vi "Rework补充.vi"() -> ()   [LabVIEW 2014]
uses:
  <vilib>/addons/database/NI_Database_API.lvlib
  <vilib>/addons/database/Connection.llb/DB Tools Open Connec (String).vi
panel:
  in  "选项卡控件":enum32{"主界面", "监控界面"}(tab)
  in  "退出":bool
  in  "RFID值":string
  in  "确定按钮":bool
  out "修改状态":string
  out "error out":errorcluster
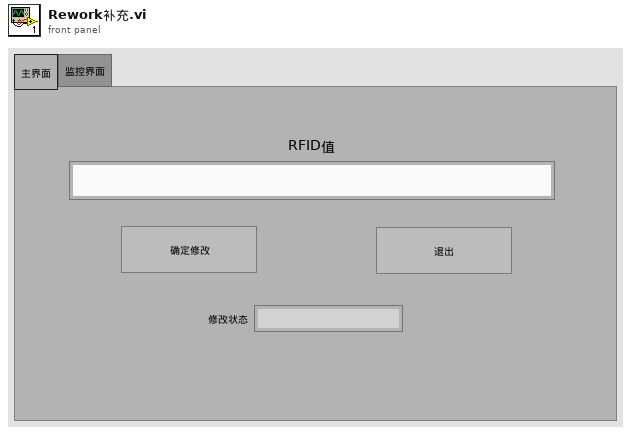
[diagram p1: front panel]
types:
  T1 = typedef "NI_Database_API.lvlib/Conn ObjectReference.ctl" = refnum<k1>
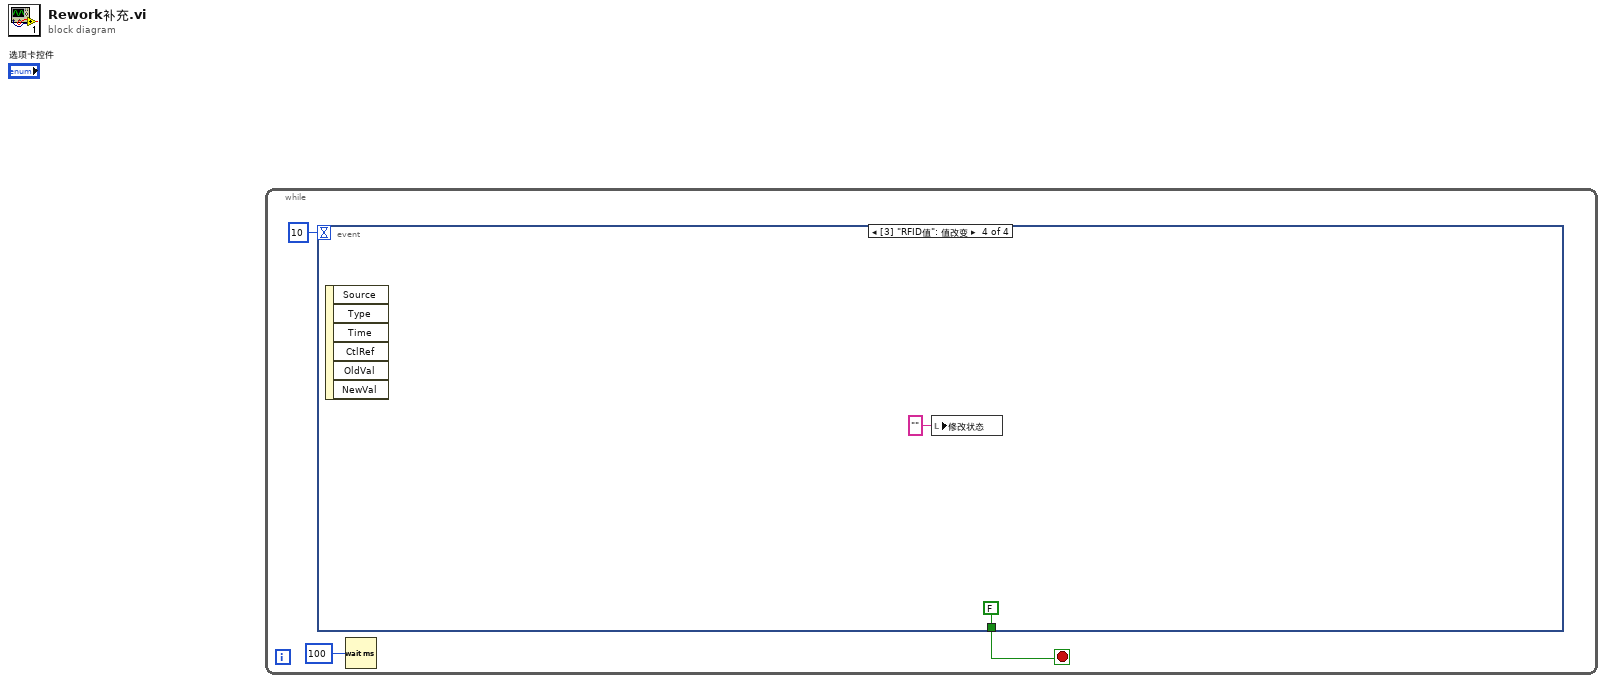
[diagram p0: block diagram]
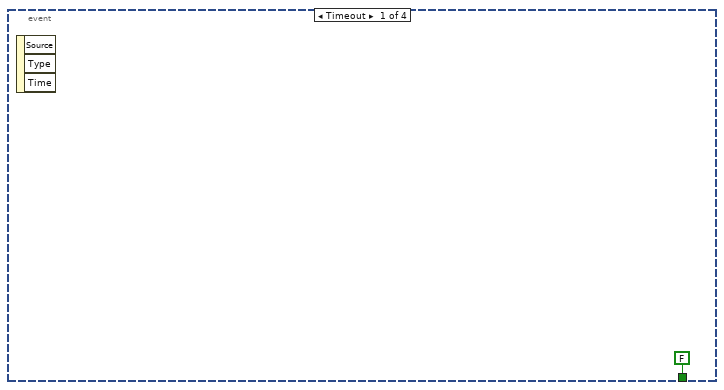
[diagram p2: hidden frame]
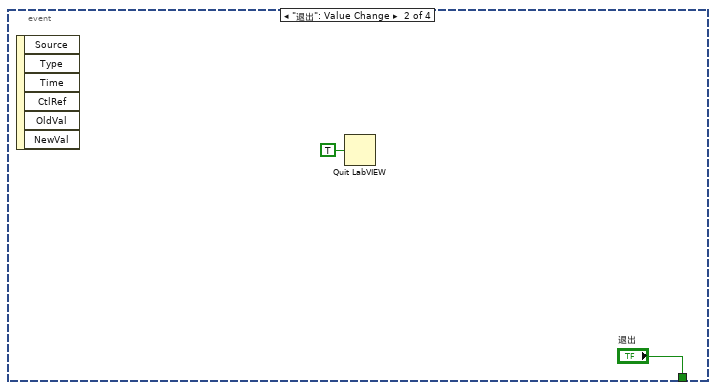
[diagram p3: hidden frame]
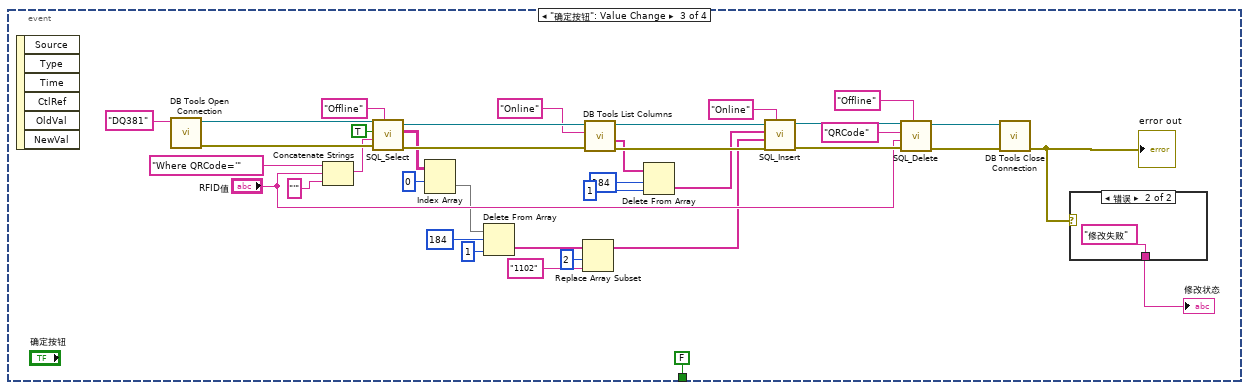
[diagram p4: hidden frame]
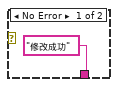
[diagram p5: hidden frame]
diagram:
  n1 = while {
    stop <- w2 stop-if-true
    n2 = event shown="[3] \"RFID值\": 值改变" {
      selector: _ -> [_ _ _ _]
      dyn-events: _ -> [_ _ _ _]
      timeout: 10 -> [_ _ _ _]
      tunnel: [FALSE ("退出") "退出" FALSE ("退出") FALSE ("退出")] -> w2
      event Timeout {
        n3 = event-data() -> ()  [unwired: 1 in, 3 out]
      }
      event "退出": Value Change {
        n4 = event-data() -> ()  [unwired: 1 in, 6 out]
        n5 = Quit LabVIEW(quit? (T)=TRUE ("退出？(T)")) -> ()
      }
      event "确定按钮": Value Change {
        n6 = event-data() -> ()  [unwired: 1 in, 6 out]
        n7 = call-poly <vilib>:"DB Tools Open Connection.vi"("connection information"="DQ381") -> ("error out"=w40:errorcluster, "connection reference"=w41:T1)  [unwired: 7 in]
        n8 = Concatenate Strings("Where QRCode='" ("查询语句"), "RFID值", "'" ("字符串")) -> (w35:string)
        n9 = call "SQL_Select.vi"("表名"="Offline", "error in (no error)"=w40, "查询语句"=w35, "查询条件"=TRUE, "connection reference"=w41) -> ("error out"=w30:errorcluster, "数据"=w17:string[][], "connection reference out"=w31:T1)  [unwired: 4 in]
        n10 = Index Array(array=w17, index (row)=0 ("索引 (行)")) -> (element=w15:string[])  [unwired: 1 in]
        n11 = Delete From Array(array=w15, length=184 ("长度"), index=1 ("索引 (行)")) -> (deleted portion=w9:string[])  [unwired: 1 out]
        n12 = Replace Array Subset(array=w9, new element="1102" ("新元素/子数组"), index=2 ("索引")) -> (w8:string[])
        n13 = call <vilib>:"DB Tools List Columns.vi"("error in (no error)"=w30, "table"="Online", "connection reference"=w31) -> ("error out"=w28:errorcluster, "columns"=w23:string[], "connection reference out"=w29:T1)  [unwired: 1 in, 1 out]
        n14 = Delete From Array(array=w23, length=184 ("长度"), index=1 ("索引")) -> (deleted portion=w20:string[])  [unwired: 1 out]
        n15 = call "SQL_Insert.vi"("表名"="Online", "error in (no error)"=w28, "值"=w8, "列名"=w20, "connection reference"=w29) -> ("error out"=w32:errorcluster, "connection reference 2"=w33:T1)  [unwired: 5 in]
        n16 = call "SQL_Delete.vi"("表名"="Offline", "error in (no error)"=w32, "值"="RFID值", "列名"="QRCode", "connection reference"=w33) -> ("error out"=w25:errorcluster, "connection reference 2"=w26:T1)  [unwired: 5 in]
        n17 = call <vilib>:"DB Tools Close Connection.vi"("error in (no error)"=w25, "connection reference"=w26) -> ("error out"=w14:errorcluster)  [unwired: 5 in]
        "error out" <- w14
        n18 = case shown="错误" w14 {
          tunnel: ["修改成功" ("修改状态") "修改失败" ("修改状态")] -> w7
          frame No Error {
          }
          frame Error {
          }
        }
        "修改状态" <- w7
      }
      event "RFID值": Value Change {
        n19 = event-data() -> ()  [unwired: 1 in, 6 out]
        n20 = local write "修改状态"("" ("修改状态")) -> ()
      }
    }
    n21 = Wait (ms)(milliseconds to wait=u32 100 ("等待时间（毫秒）")) -> ()  [unwired: 1 out]
  }
